vi "Write Numeric Scalar to Source (Base10 I32).vi"(8 "width (-)":i16, 9 "offset":i32, 10 "value":i32, 11 "error in":errorcluster) -> (1 "new offset":i32, 3 "error out":errorcluster)   [LabVIEW 2027, in "Static Errors.lvlib"]
doc: "Converts <b>value</b> into an decimal-formatted string, and writes the string to the <b>error in</b> source buffer at the specified <b>offset</b>."
uses:
  Static Errors.lvlib
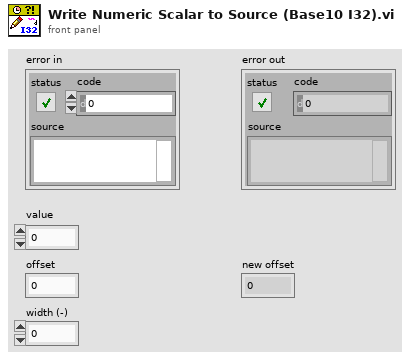
[diagram p1: front panel]
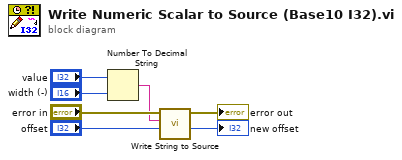
[diagram p0: block diagram]
diagram:
  n1 = Number To Decimal String(number="value", width (-)="width (-)") -> (decimal integer string=w3:string)
  n2 = call "Write String to Source.vi"("offset"="offset", "string"=w3, "error in"="error in") -> ("new offset"=→"new offset":i32, "error out"=→"error out":errorcluster)  [unwired: 7 in]
